vi "Configure Strobe Timing.vi"(0 "VISA resource name":refnum<visa-resource-name>, 1 "Strobe Timing to Configure (2:Both)":u16(ring)=2 items=["Single Strobe", "Continuous Strobe", "Both"], 2 "Continuous Strobe Rate (10 ms)":u8=10 min=1 step=1, 5 "Single Strobe High Transitional Delay Counter (1)":u16=1, 7 "Single Strobe Low Transitional Delay Counter (5)":u16=5, 9 "Continuous Strobe Base Clock Divisor (48000)":u16=48000, 11 "error in (no error)":errorcluster, 12 "Continuous Strobe Divisor (4800)":u16=4800) -> (4 "VISA resource name out":refnum<visa-resource-name>, 15 "error out":errorcluster)   [LabVIEW 2024, in "Ocean Optics 2000 4000.lvlib"]
doc: "Configures the continuous or single strobe timing or both."
uses:
  Ocean Optics 2000 4000.lvlib
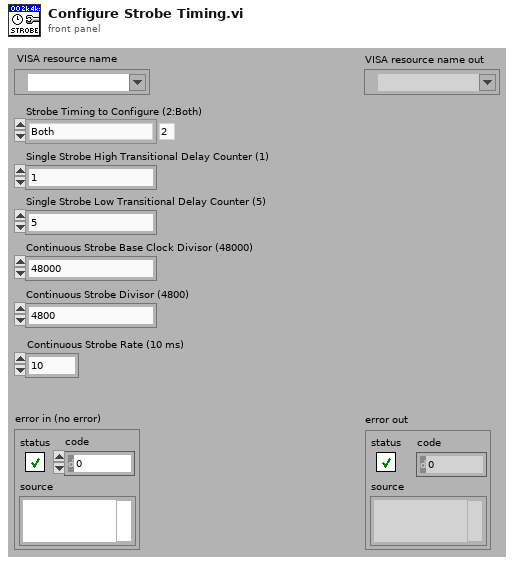
[diagram p1: front panel]
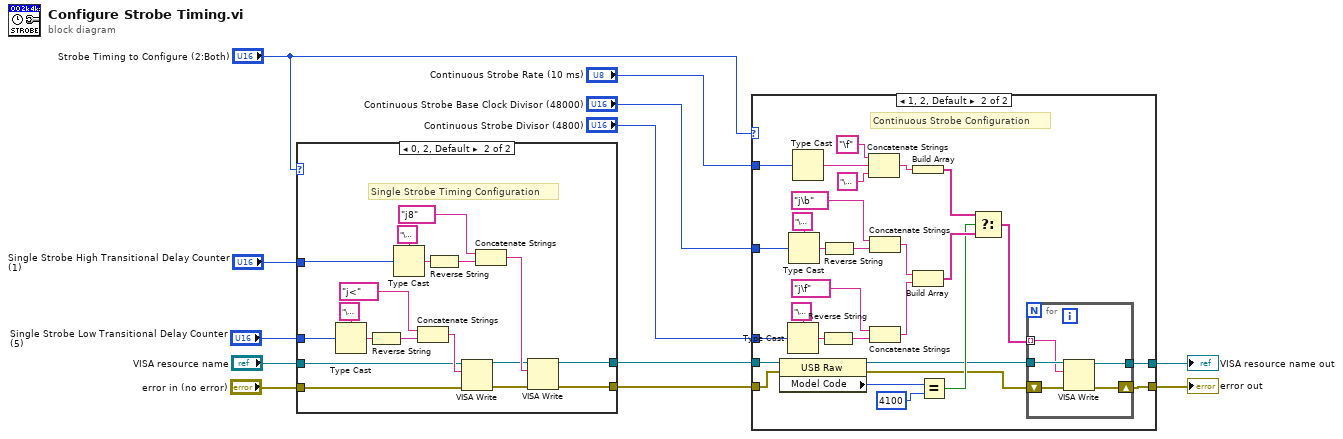
[diagram p0: block diagram]
diagram:
  n1 = case shown="0, 2, Default" "Strobe Timing to Configure (2:Both)" {
    tunnel: "Single Strobe High Transitional Delay Counter (1)" -> [_ w30]
    tunnel: "Single Strobe Low Transitional Delay Counter (5)" -> [_ w21]
    tunnel: "VISA resource name" -> [w14 w20]
    tunnel: "error in (no error)" -> [w13 w19]
    tunnel: [w14 w16] -> w6
    tunnel: [w13 w15] -> w5
    frame 1 {
      # "Single Strobe Configuration not selected"
    }
    frame 0, 2, Default {
      # "Single Strobe Timing Configuration"
      n2 = Type Cast(type="\u0000", x=w21) -> (*(type *) &x=w23:string)
      n3 = Reverse String(1:w23) -> (0:w22:string)
      n4 = Type Cast(type="\u0000", x=w30) -> (*(type *) &x=w28:string)
      n5 = Concatenate Strings("j<" ("string"), w22) -> (w26:string)
      n6 = Reverse String(1:w28) -> (0:w27:string)
      n7 = VISA Write(VISA resource name=w20, write buffer=w26, error in (no error)=w19) -> (VISA resource name out=w18:refnum<visa-resource-name>, error out=w17:errorcluster)  [unwired: 1 out]
      n8 = Concatenate Strings("j8" ("string"), w27) -> (w32:string)
      n9 = VISA Write(VISA resource name=w18, write buffer=w32, error in (no error)=w17) -> (VISA resource name out=w16:refnum<visa-resource-name>, error out=w15:errorcluster)  [unwired: 1 out]
    }
  }
  n10 = case shown="1, 2, Default" "Strobe Timing to Configure (2:Both)" {
    tunnel: "Continuous Strobe Base Clock Divisor (48000)" -> [_ w60]
    tunnel: "Continuous Strobe Divisor (4800)" -> [_ w55]
    tunnel: w6 -> [w34 w54]
    tunnel: w5 -> [w33 w53]
    tunnel: [w34 w38] -> w4
    tunnel: [w33 w37] -> w3
    tunnel: "Continuous Strobe Rate (10 ms)" -> [_ w50]
    frame 0 {
      # "Continuous strobe configuration not selected"
    }
    frame 1, 2, Default {
      # "Continuous Strobe Configuration"
      n11 = property class="USB Raw"(reference=w54, error in=w53) -> (reference out=w40:refnum<visa-resource-name>, error out=w39:errorcluster, "Model Code"=w43:u16)
      n12 = Type Cast(type="\u0000", x=w55) -> (*(type *) &x=w58:string)
      n13 = Type Cast(type="\u0000", x=w60) -> (*(type *) &x=w62:string)
      n14 = Type Cast(x=w50) -> (*(type *) &x=w48:string)  [unwired: 1 out]
      n15 = Reverse String(1:w58) -> (0:w59:string)
      n16 = Reverse String(1:w62) -> (0:w61:string)
      n17 = Concatenate Strings("\f" ("type"), w48, "\u0000" ("type")) -> (w46:string)
      n18 = Concatenate Strings("j\b" ("string"), w61) -> (w52:string)
      n19 = Concatenate Strings("j\f" ("string"), w59) -> (w51:string)
      n20 = Build Array(w46) -> (w45:string[])
      n21 = Build Array(w52, w51) -> (w44:string[])
      n22 = Equal?(x=w43, y=u16 4100) -> (x = y?=w41:bool)
      n23 = Select(t=w45, s=w41, f=w44) -> (s? t:f=w36:string[])
      n24 = for {
        tunnel: w40 -> [w68]
        tunnel: [w67] -> w38
        tunnel: w36 -> [w64] mode=indexing
        shift-right: [w65] -> w37
        shift-left: w39 -> [w66]
        n25 = VISA Write(VISA resource name=w68, write buffer=w64, error in (no error)=w66) -> (VISA resource name out=w67:refnum<visa-resource-name>, error out=w65:errorcluster)  [unwired: 1 out]
      }
    }
  }
  "VISA resource name out" <- w4
  "error out" <- w3
